vi "Make Waveforms Same Length.vi"(9 "waveform 2":waveform(dbl)={"t0"=timestamp(0 s since 1904-01-01), "dt"=0.0, "Y"=[]}, 11 "waveform 1":waveform(dbl)={"t0"=timestamp(0 s since 1904-01-01), "dt"=0.0, "Y"=[]}) -> (1 "waveform 2":waveform(dbl), 3 "waveform 1":waveform(dbl))   [LabVIEW 2022 SP3]
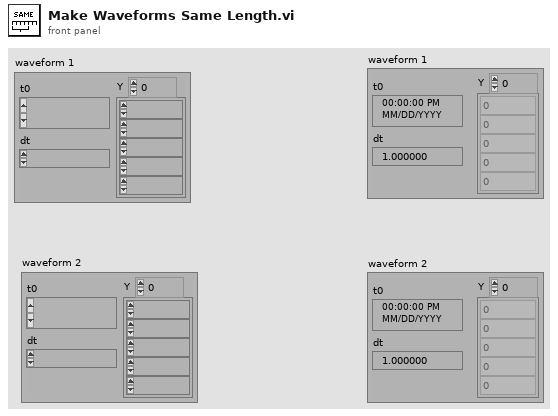
[diagram p1: front panel]
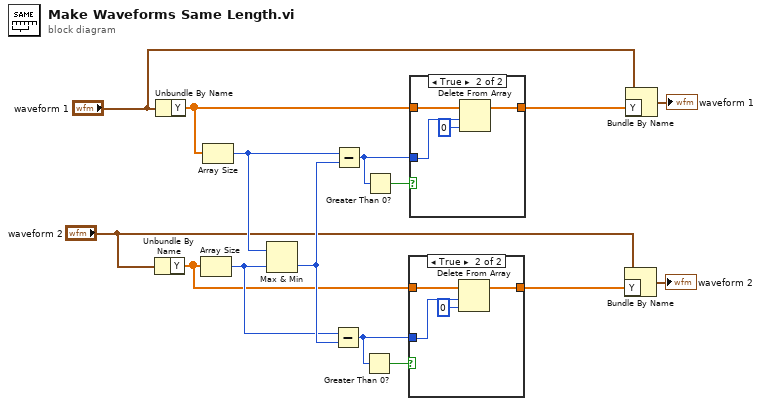
[diagram p0: block diagram]
diagram:
  n1 = Unbundle By Name("waveform 2") -> ("Y"=w3:dbl[])
  n2 = Unbundle By Name("waveform 1") -> ("Y"=w12:dbl[])
  n3 = Array Size(array=w3) -> (size(s)=w5:i32)
  n4 = Array Size(array=w12) -> (size(s)=w15:i32)
  n5 = Max & Min(x=w15, y=w5) -> (min(x,y)=w6:i32)  [unwired: 1 out]
  n6 = Subtract(x=w5, y=w6) -> (x-y=w8:i32)
  n7 = Subtract(x=w15, y=w6) -> (x-y=w13:i32)
  n8 = Greater Than 0?(x=w8) -> (x > 0?=w7:bool)
  n9 = Greater Than 0?(x=w13) -> (x > 0?=w14:bool)
  n10 = case shown="True" w7 {
    tunnel: w8 -> [_ w18]
    tunnel: w3 -> [w16 w19]
    tunnel: [w16 w20] -> w9
    frame False {
    }
    frame True {
      n11 = Delete From Array(array=w19, length=w18, index=0) -> (array with subset deleted=w20:dbl[])  [unwired: 1 out]
    }
  }
  n12 = case shown="True" w14 {
    tunnel: w13 -> [_ w23]
    tunnel: w12 -> [w21 w24]
    tunnel: [w21 w25] -> w10
    frame False {
    }
    frame True {
      n13 = Delete From Array(array=w24, length=w23, index=0) -> (array with subset deleted=w25:dbl[])  [unwired: 1 out]
    }
  }
  n14 = Bundle By Name(cluster="waveform 2", "Y"=w9) -> (→"waveform 2":waveform(dbl))
  n15 = Bundle By Name(cluster="waveform 1", "Y"=w10) -> (→"waveform 1":waveform(dbl))
